vi "UartHelper.vi"() -> ()   [LabVIEW 2012]
uses:
  <vilib>/Platform/TimedLoop/XDataNode/timing_clust.ctl
  <vilib>/Platform/TimedLoop/XDataNode/nitl_modes.ctl
  <vilib>/Platform/TimedLoop/XDataNode/wakeup.ctl
  <vilib>/event_ctls.llb/eventvkey.ctl
  <vilib>/Instr/_visa.llb/VISA Configure Serial Port (Instr).vi
  <vilib>/Platform/TimedLoop/XDataNode/XDataNode.xnode
  <vilib>/Platform/TimedLoop/XDataNode/XDNodeRunTimeDep.lvlib
panel:
  out "串口打开?":bool
  out "附加位":string="\r"
  out "文件發送":path=path "E:/ProJect/#034 串口助手/Libs/SubVi/123.txt"
  out "文件接收":path
  in  "复位计数":bool
  in  "接收计数":u32
  in  "发送计数":u32
  in  "发送数据":bool
  in  "数据发送":string
  in  "数据接收":string
  in  "清除发送":bool
  in  "清除接收":bool
  in  "循环周期":u32
  in  "循环发送":bool
  in  "文件数据源":bool
  in  "自动附加位":bool
  in  "发送模式":enum32{"ASCII", "HEX"}(radio)
  in  "接收模式":enum32{"ASCII", "HEX"}(radio)
  in  "暂停显示":bool
  in  "文件接收":bool
  in  "接收换行":bool
  in  "日志模式":bool
  in  "停止位":u32(ring)=10 items=["1"=10, "1.5"=15, "2"=20]
  in  "校验位":u16(ring) items=["None", "Odd", "Even", "Mark", "Space"]
  in  "数据位":u16(ring)=8 items=["5"=5, "6"=6, "7"=7, "8"=8]
  in  "波特率":u32(ring)=9600 items=["110"=110, "300"=300, "600"=600, "1200"=1200, "2400"=2400, "4800"=4800, "9600"=9600, "14400"=14400, "19200"=19200, "38400"=38400, "56000"=56000, "57600"=527600, "115200"=115200, "128000"=128000, "256000"=256000]
  in  "串口号":refnum<visa-resource-name>="COM1"
  in  "打开串口":bool
  # "串口设置"
  # "接收设置"
  # "发送设置"
  # "ms"
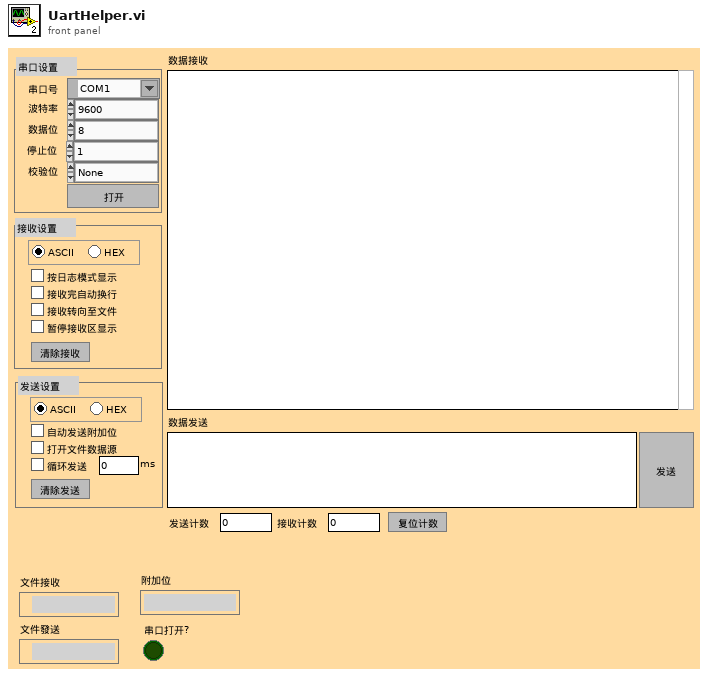
[diagram p1: front panel]
types:
  T1 = typedef "XDNodeRunTimeDep.lvlib/timing_clust.ctl" = cluster{"Expected End [f-1]":u64, "Actual End [f-1]":u64, "Finished Late? [f-1]":bool, "Expected End [i-1]":u64, "Actual End [i-1]":u64, "Finished Late? [i-1]":bool, "Expected Start [i]":u64, "Actual Start [i]":u64, "Expected Start [f]":u64, "Actual Start [f]":u64, "Source Name":string, "Structure Name":string, "Period":i64, "Deadline":i64, "Offset":i64, "Start":i64, "Priority":i32, "Timeout":i32, "Mode":T2, "Wakeup Reason":T3, "Error":errorcluster, "Source Type":string, "Secondary Source Type":string, "Global End Time":u64, "Global Start Time":u64, "Frame Duration":u64, "Iteration Duration":u64, "Assigned CPU":i32, "I/O Scan Engine Mode":u32}
  T2 = typedef "XDNodeRunTimeDep.lvlib/nitl_modes.ctl" = enum32{"No Change", "Process missed periods, maintain original phase", "Discard missed periods, maintain original phase", "Process missed periods, ignore original phase", "Discard missed periods, ignore original phase"}
  T3 = typedef "XDNodeRunTimeDep.lvlib/wakeup.ctl" = enum32{"Normal", "Aborted", "Asynchronous wakeup", "Timing source error", "Timed loop error", "Timeout"}
  T4 = enum8{"Enabled", "Disabled", "Disabled and Grayed Out"}
  T5 = typedef "eventvkey.ctl" = enum16{"ASCII", "Enter", "Return", "Shift", "Ctrl", "Alt", "Cmd", "Opt", "Caps", "NumLock", "Clear", "Break", "Up", "Down", "Left", "Right", "Insert", "Delete", "Home", "End", "PageUp", "PageDown", "Escape", "Help", "Pause", "ScrollLock", "F1", "F2", "F3", "F4", "F5", "F6", "F7", "F8", "F9", "F10", "F11", "F12", "F13", "F14", "F15", "F16", "F17", "F18", "F19", "F20", "F21", "F22", "F23", "F24", "Play", "VolumeUp", "VolumeDown", "Mute", "Two Byte Char"}
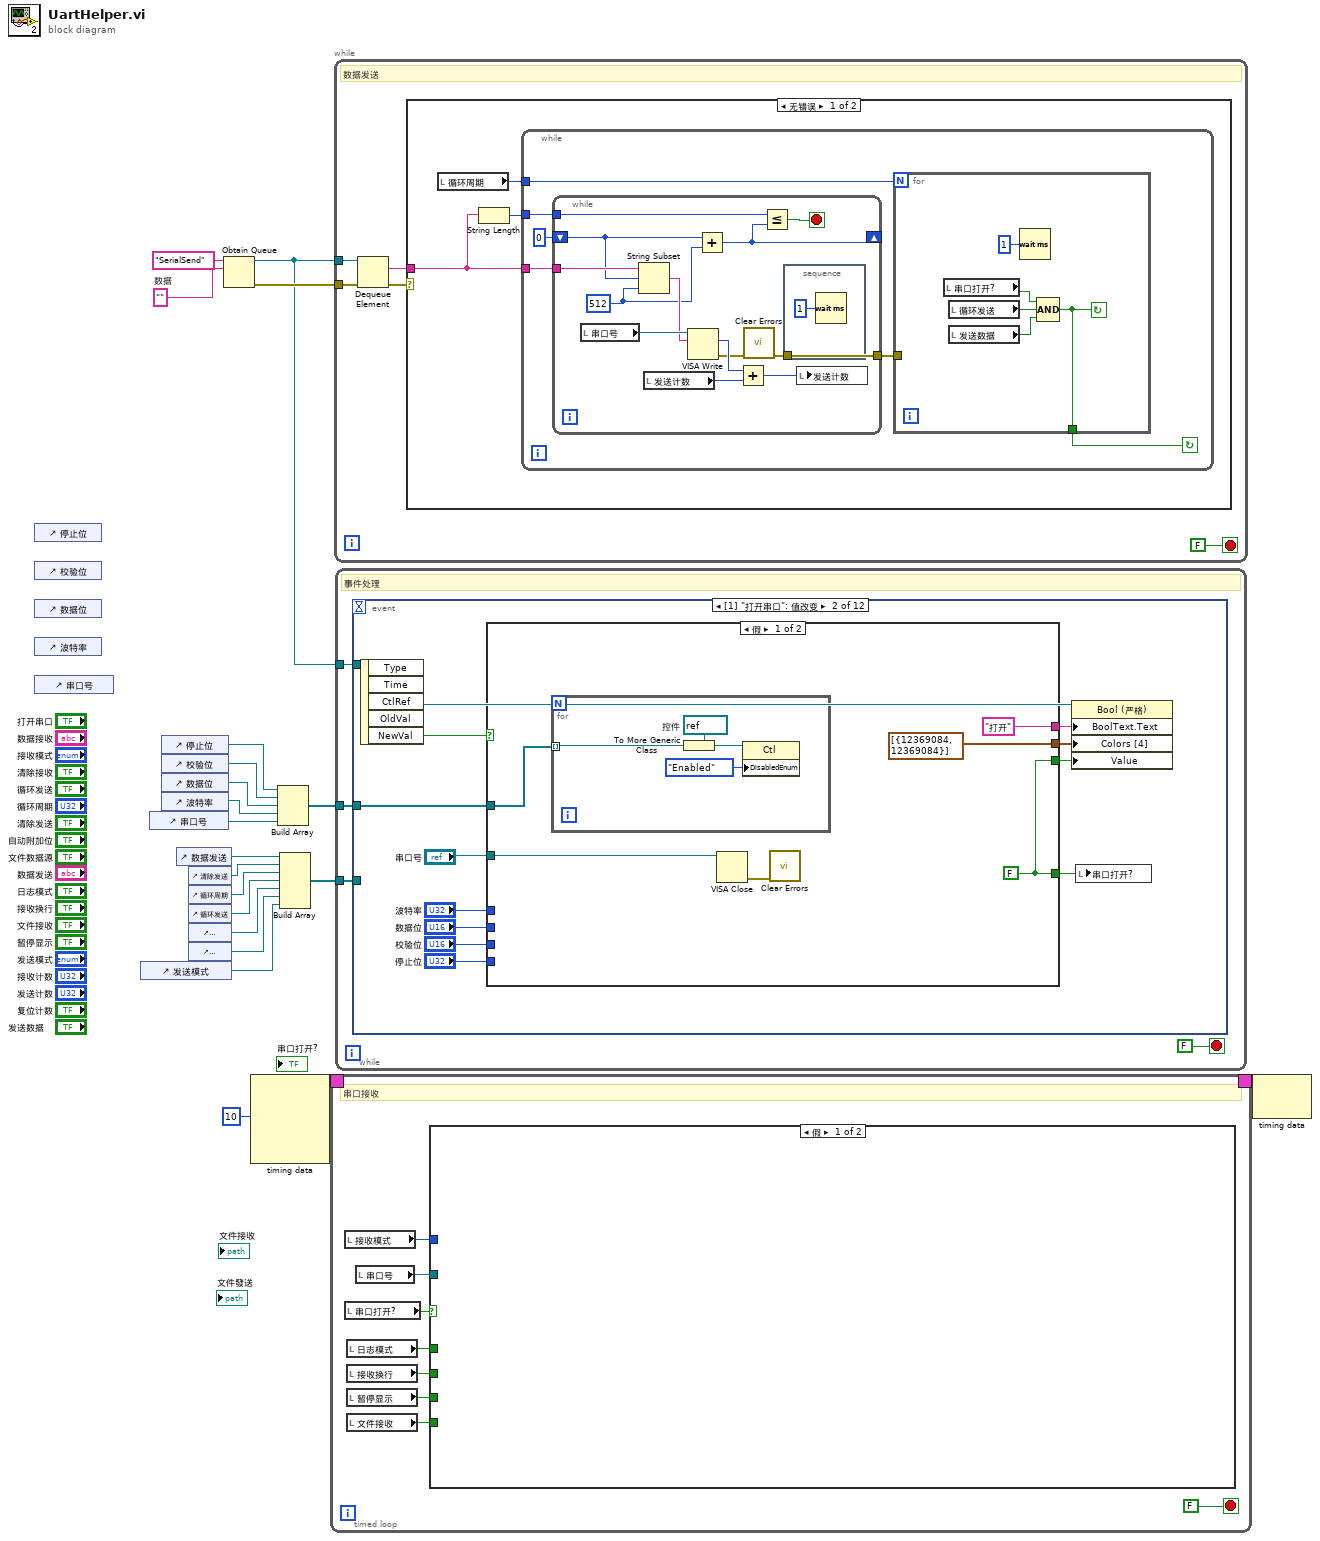
[diagram p0: block diagram]
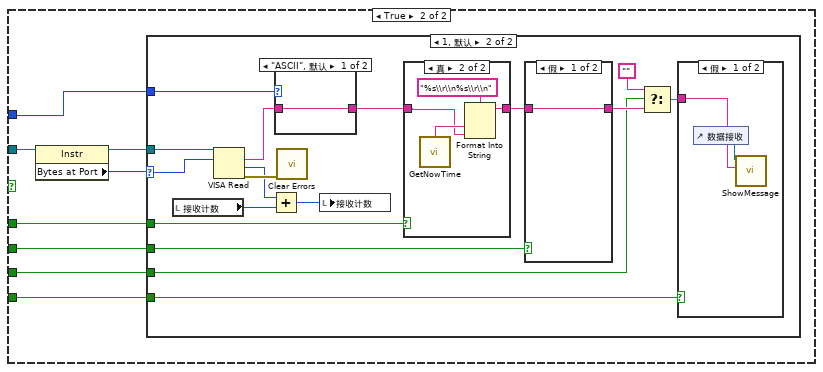
[diagram p3: hidden frame]
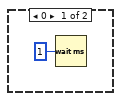
[diagram p4: hidden frame]
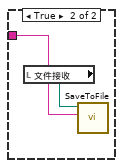
[diagram p5: hidden frame]
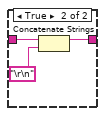
[diagram p6: hidden frame]
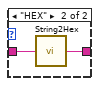
[diagram p8: hidden frame]
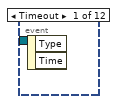
[diagram p9: hidden frame]
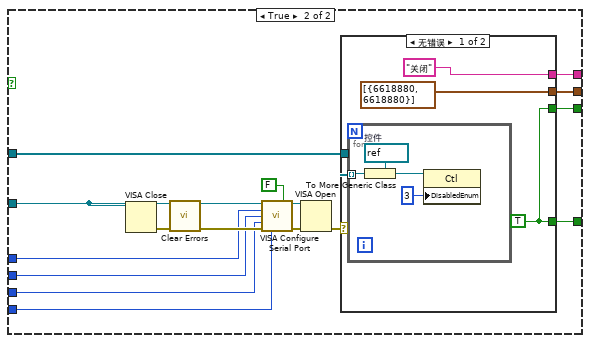
[diagram p10: hidden frame]
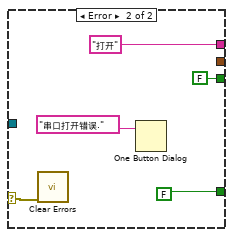
[diagram p11: hidden frame]
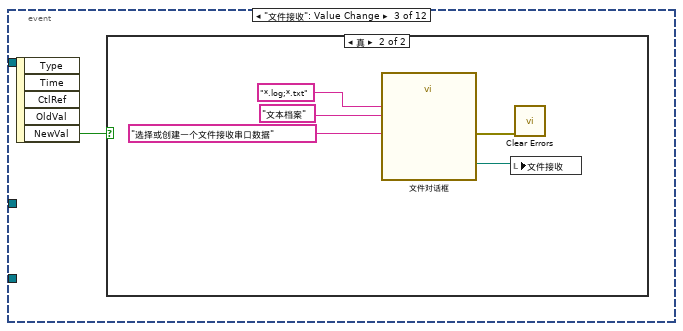
[diagram p12: hidden frame]
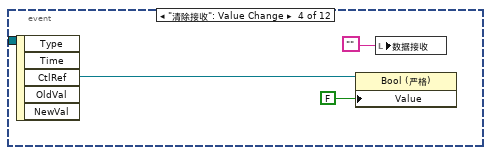
[diagram p14: hidden frame]
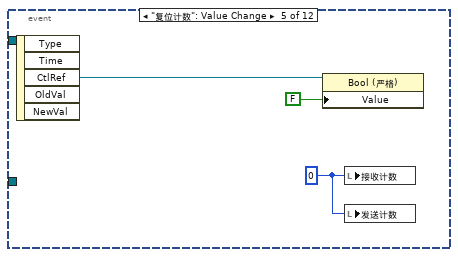
[diagram p15: hidden frame]
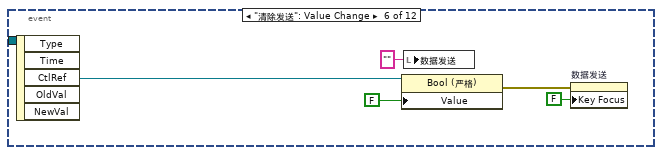
[diagram p16: hidden frame]
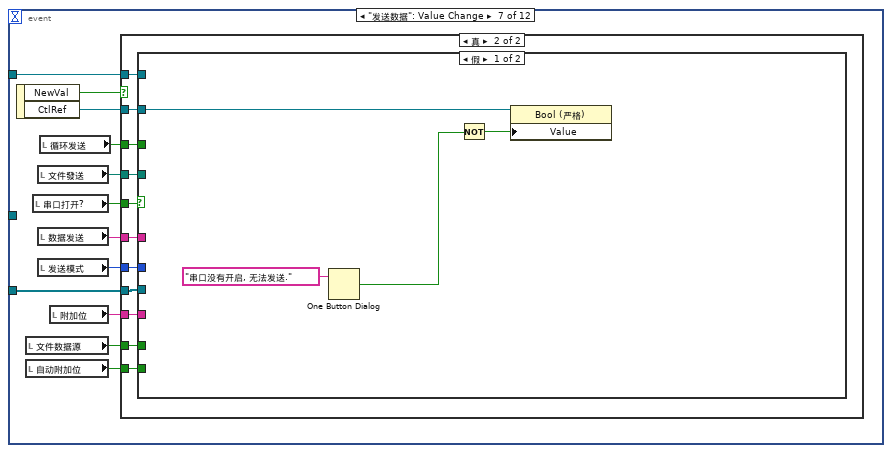
[diagram p17: hidden frame]
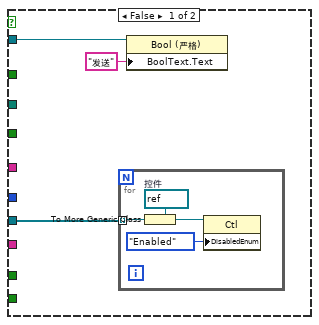
[diagram p18: hidden frame]
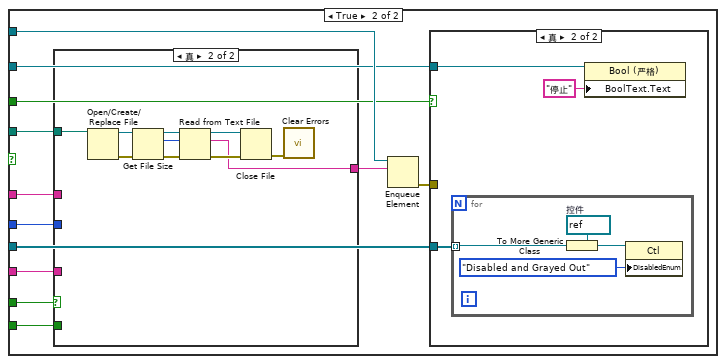
[diagram p19: hidden frame]
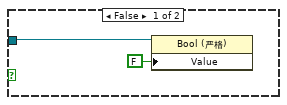
[diagram p20: hidden frame]
diagram:
  w16 = ""  # 数据
  n1 = control-ref of="停止位"() -> ()  [unwired: 1 out]
  n2 = control-ref of="校验位"() -> ()  [unwired: 1 out]
  n3 = control-ref of="数据位"() -> ()  [unwired: 1 out]
  n4 = control-ref of="波特率"() -> ()  [unwired: 1 out]
  n5 = control-ref of="串口号"() -> ()  [unwired: 1 out]
  n6 = control-ref of="发送模式"() -> (w8:refnum<vi>)
  n7 = control-ref of="串口号"() -> (w6:refnum<vi>)
  n8 = control-ref of="停止位"() -> (w2:refnum<vi>)
  n9 = control-ref of="校验位"() -> (w3:refnum<vi>)
  n10 = control-ref of="数据位"() -> (w4:refnum<vi>)
  n11 = control-ref of="波特率"() -> (w5:refnum<vi>)
  n12 = control-ref of="数据发送"() -> (w14:refnum<vi>)
  n13 = control-ref of="清除发送"() -> (w13:refnum<vi>)
  n14 = control-ref of="循环周期"() -> (w12:refnum<vi>)
  n15 = control-ref of="循环发送"() -> (w11:refnum<vi>)
  n16 = control-ref of="文件数据源"() -> (w10:refnum<vi>)
  n17 = control-ref of="自动附加位"() -> (w9:refnum<vi>)
  n18 = Obtain Queue(name (unnamed)="SerialSend" ("名称（未命名）"), element data type=w16) -> (queue out=w15:refnum<queue>, error out=w18:errorcluster)  [unwired: 3 in, 1 out]
  n19 = node-c288(i64 10 ("周期")) -> (w21:T1)  [unwired: 3 in]
  n20 = Build Array(w2, w3, w4, w5, w6) -> (w1:refnum<vi>[])
  n21 = Build Array(w14, w13, w12, w11, w10, w9, w8) -> (w7:refnum<vi>[])
  n22 = timed-loop "接收" {
    timing: w21 -> [_]
    timing-out: [_] -> w20
    stop <- FALSE stop-if-true
    # "串口接收"
    n23 = local read "接收模式"() -> (w27:enum32{"ASCII", "HEX"})
    n24 = local read "串口打开?"() -> (w26:bool)
    n25 = local read "日志模式"() -> (w25:bool)
    n26 = local read "接收换行"() -> (w24:bool)
    n27 = local read "暂停显示"() -> (w23:bool)
    n28 = local read "文件接收"() -> (w22:bool)
    n29 = local read "串口号"() -> (w28:refnum<visa-resource-name>)
    n30 = case shown="假" w26 {
      tunnel: w28 -> [_ w37]
      tunnel: w27 -> [_ w35]
      tunnel: w25 -> [_ w34]
      tunnel: w24 -> [_ w33]
      tunnel: w23 -> [_ w32]
      tunnel: w22 -> [_ w31]
      frame False {
      }
      frame True {
        n31 = property class="Instr"(reference=w37) -> (reference out=w36:refnum<visa-resource-name>, "Bytes at Port"=w30:u32)  [unwired: 1 in, 1 out]
        n32 = case shown="1, 默认" w30 {
          selector: w30 -> [_ w39]
          tunnel: w36 -> [_ w55]
          tunnel: w35 -> [_ w54]
          tunnel: w34 -> [_ w48]
          tunnel: w33 -> [_ w46]
          tunnel: w32 -> [_ w43]
          tunnel: w31 -> [_ w41]
          frame 0 {
            n33 = Wait (ms)(milliseconds to wait=u32 1 ("等待时间（毫秒）")) -> ()  [unwired: 1 out]
          }
          frame 1, Default {
            n34 = local read "接收计数"() -> (w50:u32)
            n35 = VISA Read(VISA resource name=w55, byte count=w39) -> (read buffer=w53:string, return count=w51:u32, error out=w52:errorcluster)  [unwired: 1 in, 1 out]
            n36 = Add(x=w51, y=w50) -> (x+y=w49:u32)
            n37 = case shown="\"ASCII\", 默认" w54 {
              tunnel: w53 -> [w69 w71]
              tunnel: [w69 w70] -> w47
              frame "ASCII", Default {
              }
              frame "HEX" {
                n38 = call "String2Hex.vi"("String"=w71) -> ("Hex"=w70:string)
              }
            }
            n39 = call <vilib>:"Clear Errors.vi"("error in (no error)"=w52) -> ()  [unwired: 6 in, 1 out]
            n40 = local write "接收计数"(w49) -> ()
            n41 = case shown="真" w48 {
              tunnel: w47 -> [w64 w66]
              tunnel: [w64 w68] -> w45
              frame False {
              }
              frame True {
                n42 = call "GetNowTime.vi"() -> ("NowTime"=w67:string)
                n43 = Format Into String(format string="%s\\r\\n%s\\r\\n" ("格式字符串"), w67, w66) -> (resulting string=w68:string)  [unwired: 2 in, 1 out]
              }
            }
            n44 = case shown="假" w46 {
              tunnel: w45 -> [w60 w63]
              tunnel: [w60 w61] -> w44
              frame False {
              }
              frame True {
                n45 = Concatenate Strings(w63, "\r\n") -> (w61:string)
              }
            }
            n46 = Select(t="", s=w43, f=w44) -> (s? t:f=w40:string)
            n47 = case shown="假" w41 {
              tunnel: w40 -> [w56 w59]
              frame False {
                n48 = control-ref of="数据接收"() -> (w57:refnum<vi>)
                n49 = call "ShowMessage.vi"("字符串"=w56, "Str引用句柄"=w57) -> ()  [unwired: 10 in]
              }
              frame True {
                n50 = local read "文件接收"() -> (w58:path)
                n51 = call "SaveToFile.vi"("字符串"=w59, "路径"=w58) -> ()  [unwired: 10 in]
              }
            }
          }
        }
      }
    }
  }
  n52 = while {
    tunnel: w15 -> [w75]
    tunnel: w18 -> [w74]
    stop <- FALSE stop-if-true
    # "数据发送"
    n53 = Dequeue Element(queue=w75, error in (no error)=w74) -> (element=w76:string, error out=w77:errorcluster)  [unwired: 1 in, 2 out]
    n54 = case shown="无错误" w77 {
      tunnel: w76 -> [w80 _]
      frame No Error {
        n55 = local read "循环周期"() -> (w81:u32)
        n56 = String Length(string=w80) -> (length=w79:i32)
        n57 = while {
          tunnel: w80 -> [w87]
          tunnel: w81 -> [w86]
          tunnel: w79 -> [w82]
          stop <- w84 continue-if-true
          n58 = while {
            tunnel: [w88] -> w85
            tunnel: w87 -> [w95]
            shift-right: [w90] -> _
            shift-left: 0 -> [w93]
            tunnel: w82 -> [w91]
            stop <- w89 stop-if-true
            w92 = 512 ("长度（剩余）")
            n59 = local read "串口号"() -> (w100:refnum<visa-resource-name>)
            n60 = String Subset(string=w95, offset (0)=w93, length (rest)=w92) -> (substring=w94:string)
            n61 = local read "发送计数"() -> (w99:u32)
            n62 = VISA Write(VISA resource name=w100, write buffer=w94) -> (return count=w98:u32, error out=w97:errorcluster)  [unwired: 1 in, 1 out]
            n63 = Add(x=w93, y=w92) -> (x+y=w90:i32)
            n64 = Add(x=w98, y=w99) -> (x+y=w96:u32)
            n65 = call <vilib>:"Clear Errors.vi"("error in (no error)"=w97) -> ("error out"=w88:errorcluster)  [unwired: 6 in]
            n66 = Less Or Equal?(x=w91, y=w90) -> (x <= y?=w89:bool)
            n67 = stacked-sequence {
              tunnel: w88 -> [_]
              frame #0 {
                n68 = Wait (ms)(milliseconds to wait=u32 1 ("等待时间（毫秒）")) -> ()  [unwired: 1 out]
              }
            }
            n69 = local write "发送计数"(w96) -> ()
          }
          n70 = for {
            N: w86 -> [_]
            tunnel: w85 -> [_]
            tunnel: [w103] -> w84
            stop <- w103 continue-if-true
            n71 = local read "串口打开?"() -> (w102:bool)
            n72 = local read "循环发送"() -> (w105:bool)
            n73 = local read "发送数据"() -> (w104:bool)
            n74 = Wait (ms)(milliseconds to wait=u32 1 ("等待时间（毫秒）")) -> ()  [unwired: 1 out]
            n75 = Compound Arithmetic op=AND(w102, w105, w104) -> (w103:bool)
          }
        }
      }
      frame Error {
      }
    }
  }
  n76 = while {
    tunnel: w15 -> [w109]
    tunnel: w7 -> [w108]
    tunnel: w1 -> [w107]
    stop <- FALSE stop-if-true
    # "事件处理"
    n77 = event shown="[1] \"打开串口\": 值改变" {
      selector: _ -> [_ _ _ _ _ _ _ _ _ _ _ _]
      dyn-events: _ -> [_ _ _ _ _ _ _ _ _ _ _ _]
      timeout: _ -> [_ _ _ _ _ _ _ _ _ _ _ _]
      tunnel: w109 -> [_ _ _ _ _ _ w185 _ _ _ _ _]
      tunnel: w108 -> [_ _ _ _ _ _ w179 _ _ _ _ _]
      tunnel: w107 -> [_ w116 _ _ _ _ _ _ _ _ _ _]
      event Timeout {
        n78 = event-data() -> ()  [unwired: 1 in, 2 out]
      }
      event "打开串口": Value Change {
        n79 = event-data() -> ("CtlRef"=w121:refnum<vi>, "NewVal"=w122:bool)  [unwired: 1 in, 3 out]
        n80 = case shown="假" w122 {
          tunnel: ["打开" w148] -> w120
          tunnel: [cluster{u32, u32}[] [{12369084, 12369084}] w147] -> w119
          tunnel: [w125 w145] -> w118
          tunnel: [w125 w144] -> w117
          tunnel: w116 -> [w124 w143]
          tunnel: "串口号" -> [w123 w133]
          tunnel: "波特率" -> [_ w140]
          tunnel: "数据位" -> [_ w138]
          tunnel: "校验位" -> [_ w137]
          tunnel: "停止位" -> [_ w136]
          frame False {
            w125 = FALSE
            n81 = for {
              tunnel: w124 -> [w132] mode=indexing
              w131 = refnum<vi> refnum  # 控件
              n82 = To More Generic Class(target class=w131, reference=w132) -> (generic class reference=w130:refnum<vi>)
              n83 = property class="Ctl"(reference=w130, "DisabledEnum"=T4."Enabled" ("禁用")) -> ()  [unwired: 1 in, 2 out]
            }
            n84 = VISA Close(VISA resource name=w123) -> (error out=w126:errorcluster)  [unwired: 1 in]
            n85 = call <vilib>:"Clear Errors.vi"("error in (no error)"=w126) -> ()  [unwired: 6 in, 1 out]
          }
          frame True {
            n86 = VISA Close(VISA resource name=w133) -> (error out=w134:errorcluster)  [unwired: 1 in]
            n87 = call <vilib>:"Clear Errors.vi"("error in (no error)"=w134) -> ("error out"=w141:errorcluster)  [unwired: 6 in]
            n88 = call-poly "VISA Configure Serial Port"("VISA resource name"=w133, "Enable Termination\nChar (T)"=FALSE ("Enable Termination\nChar (T)"), "baud rate (9600)"=w140, "data bits (8)"=w138, "parity (0:none)"=w137, "error in (no error)"=w141, "stop bits (10: 1 bit)"=w136) -> ("VISA resource name out"=w135:refnum<visa-resource-name>, "error out"=w142:errorcluster)  [unwired: 7 in]
            n89 = VISA Open(error in (no error)=w142, VISA resource name=w135) -> (error out=w146:errorcluster)  [unwired: 3 in, 1 out]
            n90 = case shown="无错误" w146 {
              selector: w146 -> [_ w160]
              tunnel: ["关闭" "打开"] -> w148
              tunnel: [cluster{u32, u32}[] [{6618880, 6618880}] _] -> w147
              tunnel: [w150 FALSE] -> w145
              tunnel: [w150 FALSE] -> w144
              tunnel: w143 -> [w149 _]
              frame No Error {
                w150 = TRUE
                n91 = for {
                  tunnel: w149 -> [w156] mode=indexing
                  w155 = refnum<vi> refnum  # 控件
                  n92 = To More Generic Class(target class=w155, reference=w156) -> (generic class reference=w154:refnum<vi>)
                  n93 = property class="Ctl"(reference=w154, "DisabledEnum"=3) -> ()  [unwired: 1 in, 2 out]
                }
              }
              frame Error {
                n94 = call <vilib>:"Clear Errors.vi"("error in (no error)"=w160) -> ()  [unwired: 6 in, 1 out]
                n95 = One Button Dialog(message="串口打开错误.") -> ()  [unwired: 1 in, 1 out]
              }
            }
          }
        }
        n96 = property class="Bool (严格)"(reference=w121, "BoolText.Text"=w120, "Colors [4]"=w119, "Value"=w117) -> ()  [unwired: 1 in, 2 out]
        n97 = local write "串口打开?"(w118) -> ()
      }
      event "文件接收": Value Change {
        n98 = event-data() -> ("NewVal"=w162:bool)  [unwired: 1 in, 4 out]
        n99 = case shown="真" w162 {
          frame False {
          }
          frame True {
            n100 = call "文件对话框"("prompt"="选择或创建一个文件接收串口数据", "pattern (all files)"="*.log;*.txt", "pattern label"="文本档案") -> ("selected path"=w167:path, "error out"=w165:errorcluster)  [unwired: 9 in, 2 out]
            n101 = local write "文件接收"(w167) -> ()
            n102 = call <vilib>:"Clear Errors.vi"("error in (no error)"=w165) -> ()  [unwired: 6 in, 1 out]
          }
        }
      }
      event "清除接收": Value Change {
        n103 = event-data() -> ("CtlRef"=w169:refnum<vi>)  [unwired: 1 in, 4 out]
        n104 = property class="Bool (严格)"(reference=w169, "Value"=FALSE) -> ()  [unwired: 1 in, 2 out]
        n105 = local write "数据接收"("") -> ()
      }
      event "复位计数": Value Change {
        w173 = 0
        n106 = event-data() -> ("CtlRef"=w172:refnum<vi>)  [unwired: 1 in, 4 out]
        n107 = property class="Bool (严格)"(reference=w172, "Value"=FALSE) -> ()  [unwired: 1 in, 2 out]
        n108 = local write "接收计数"(w173) -> ()
        n109 = local write "发送计数"(w173) -> ()
      }
      event "清除发送": Value Change {
        n110 = event-data() -> ("CtlRef"=w177:refnum<vi>)  [unwired: 1 in, 4 out]
        n111 = property class="Bool (严格)"(reference=w177, "Value"=FALSE) -> (error out=w175:errorcluster)  [unwired: 1 in, 1 out]
        n112 = local write "数据发送"("" ("数据发送")) -> ()
        n113 = property on="数据发送" class="Str"(error in=w175, "Key Focus"=FALSE ("键选中")) -> ()  [unwired: 1 in, 2 out]
      }
      event "发送数据": Value Change {
        n114 = event-data() -> ("NewVal"=w180:bool, "CtlRef"=w182:refnum<vi>)  [unwired: 1 in]
        n115 = local read "文件数据源"() -> (w184:bool)
        n116 = local read "自动附加位"() -> (w183:bool)
        n117 = local read "串口打开?"() -> (w188:bool)
        n118 = local read "文件發送"() -> (w186:path)
        n119 = local read "数据发送"() -> (w189:string)
        n120 = local read "发送模式"() -> (w190:enum32{"ASCII", "HEX"})
        n121 = local read "循环发送"() -> (w181:bool)
        n122 = local read "附加位"() -> (w187:string)
        n123 = case shown="真" w180 {
          tunnel: w190 -> [_ w208]
          tunnel: w189 -> [_ w207]
          tunnel: w188 -> [_ w206]
          tunnel: w187 -> [_ w205]
          tunnel: w186 -> [_ w204]
          tunnel: w185 -> [_ w203]
          tunnel: w184 -> [_ w202]
          tunnel: w183 -> [_ w201]
          tunnel: w182 -> [w193 w200]
          tunnel: w181 -> [_ w199]
          tunnel: w179 -> [w191 w198]
          frame False {
            n124 = for {
              tunnel: w191 -> [w197] mode=indexing
              w196 = refnum<vi> refnum  # 控件
              n125 = To More Generic Class(target class=w196, reference=w197) -> (generic class reference=w195:refnum<vi>)
              n126 = property class="Ctl"(reference=w195, "DisabledEnum"=T4."Enabled" ("禁用")) -> ()  [unwired: 1 in, 2 out]
            }
            n127 = property class="Bool (严格)"(reference=w193, "BoolText.Text"="发送" ("布尔文本.文本")) -> ()  [unwired: 1 in, 2 out]
          }
          frame True {
            n128 = case shown="假" w206 {
              tunnel: w208 -> [_ w224]
              tunnel: w207 -> [_ w223]
              tunnel: w205 -> [_ w222]
              tunnel: w202 -> [_ w221]
              tunnel: w204 -> [_ w220]
              tunnel: w203 -> [_ w218]
              tunnel: w201 -> [_ w219]
              tunnel: w200 -> [w211 w214]
              tunnel: w199 -> [_ w216]
              tunnel: w198 -> [_ w213]
              frame False {
                n129 = One Button Dialog(message="串口没有开启, 无法发送." ("消息")) -> (true=w209:bool)  [unwired: 1 in]
                n130 = Not(x=w209) -> (.not. x?=w210:bool)
                n131 = property class="Bool (严格)"(reference=w211, "Value"=w210) -> ()  [unwired: 1 in, 2 out]
              }
              frame True {
                n132 = case shown="真" w221 {
                  tunnel: w224 -> [w239 _]
                  tunnel: w223 -> [w238 _]
                  tunnel: w222 -> [w236 _]
                  tunnel: w220 -> [_ w251]
                  tunnel: [w235 w247] -> w217
                  tunnel: w219 -> [w234 _]
                  frame False {
                    n133 = case shown="\"HEX\"" w239 {
                      tunnel: w238 -> [w244 w246]
                      tunnel: [w244 w245] -> w237
                      frame "ASCII", Default {
                      }
                      frame "HEX" {
                        n134 = call "Hex2String.vi"("Hex"=w246) -> ("String"=w245:string)
                      }
                    }
                    n135 = case shown="真" w234 {
                      tunnel: w237 -> [w240 w243]
                      tunnel: w236 -> [_ w242]
                      tunnel: [w240 w241] -> w235
                      frame False {
                      }
                      frame True {
                        n136 = Concatenate Strings(w243, w242) -> (w241:string)
                      }
                    }
                  }
                  frame True {
                    n137 = Open/Create/Replace File(file path (use dialog)=w251) -> (refnum out=w255:refnum<file>, error out=w256:errorcluster)  [unwired: 5 in, 1 out]
                    n138 = Get File Size(file=w255, error in=w256) -> (refnum out=w250:refnum<file>, size (in bytes)=w248:i64, 0:w249:errorcluster)
                    n139 = Read from Text File(file (use dialog)=w250, count=w248, error in=w249) -> (refnum out=w253:refnum<file>, text=w247:string, error out=w254:errorcluster)  [unwired: 1 in, 1 out]
                    n140 = Close File(refnum=w253, error in=w254) -> (error out=w252:errorcluster)  [unwired: 1 out]
                    n141 = call <vilib>:"Clear Errors.vi"("error in (no error)"=w252) -> ()  [unwired: 6 in, 1 out]
                  }
                }
                n142 = Enqueue Element(queue=w218, element=w217) -> (error out=w215:errorcluster)  [unwired: 2 in, 2 out]
                n143 = case shown="真" w216 {
                  tunnel: w214 -> [w226 w229]
                  tunnel: w215 -> [_ _]
                  tunnel: w213 -> [_ w227]
                  frame False {
                    n144 = property class="Bool (严格)"(reference=w226, "Value"=FALSE ("值")) -> ()  [unwired: 1 in, 2 out]
                  }
                  frame True {
                    n145 = for {
                      tunnel: w227 -> [w233] mode=indexing
                      w232 = refnum<vi> refnum  # 控件
                      n146 = To More Generic Class(target class=w232, reference=w233) -> (generic class reference=w231:refnum<vi>)
                      n147 = property class="Ctl"(reference=w231, "DisabledEnum"=T4."Disabled and Grayed Out" ("禁用")) -> ()  [unwired: 1 in, 2 out]
                    }
                    n148 = property class="Bool (严格)"(reference=w229, "BoolText.Text"="停止" ("布尔文本.文本")) -> ()  [unwired: 1 in, 2 out]
                  }
                }
              }
            }
          }
        }
      }
      event "文件数据源": Value Change {
        n149 = event-data() -> ("CtlRef"=w257:refnum<vi>, "NewVal"=w258:bool)  [unwired: 1 in, 3 out]
        n150 = case shown="假" w258 {
          tunnel: w257 -> [_ w260]
          frame False {
            n151 = property on="数据发送" class="Str"("DisabledEnum"=T4."Enabled" ("禁用")) -> ()  [unwired: 2 in, 2 out]
          }
          frame True {
            n152 = call "文件对话框2"("prompt"="选择一个文件进行发送.") -> ("selected path"=w261:path, "exists"=w262:bool, "error out"=w263:errorcluster)  [unwired: 11 in, 1 out]
            n153 = case shown="无错误" w263 {
              selector: w263 -> [_ w272]
              tunnel: w262 -> [w267 _]
              tunnel: w261 -> [w266 _]
              tunnel: w260 -> [w265 _]
              frame No Error {
                n154 = case shown="真" w267 {
                  selector: w267 -> [w268 _]
                  tunnel: w266 -> [_ w271]
                  tunnel: w265 -> [w269 _]
                  frame False {
                    n155 = property class="Bool (严格)"(reference=w269, "Value"=w268) -> ()  [unwired: 1 in, 2 out]
                  }
                  frame True {
                    n156 = local write "文件發送"(w271) -> ()
                    n157 = property on="数据发送" class="Str"("DisabledEnum"=T4."Disabled and Grayed Out" ("禁用")) -> ()  [unwired: 2 in, 2 out]
                  }
                }
              }
              frame Error {
                n158 = call <vilib>:"Clear Errors.vi"("error in (no error)"=w272) -> ()  [unwired: 6 in, 1 out]
              }
            }
          }
        }
      }
      event "自动附加位": Value Change {
        n159 = event-data() -> ("NewVal"=w273:bool)  [unwired: 1 in, 4 out]
        n160 = case shown="真" w273 {
          frame False {
          }
          frame True {
            n161 = call "AddMessage.vi"() -> ("字符串"=→"附加位":string)
          }
        }
      }
      event "发送模式": Value Change {
        n162 = event-data() -> ("NewVal"=w277:enum32{"ASCII", "HEX"})  [unwired: 1 in, 4 out]
        n163 = local read "数据发送"() -> (w276:string)
        n164 = case shown="\"HEX\"" w277 {
          tunnel: w276 -> [w279 w281]
          tunnel: [w278 w280] -> w275
          frame "ASCII", Default {
            n165 = call "Hex2String.vi"("Hex"=w279) -> ("String"=w278:string)
          }
          frame "HEX" {
            n166 = call "String2Hex.vi"("String"=w281) -> ("Hex"=w280:string)
          }
        }
        n167 = local write "数据发送"(w275) -> ()
      }
      event "数据发送": Key Down? {
        # "输入过滤, 当HEX模式时无法输入十六进制以外的字符"
        n168 = event-data() -> ("Char"=w286:i16, "VKey"=w284:T5)  [unwired: 1 in, 7 out]
        n169 = local read "发送模式"() -> (w282:enum32{"ASCII", "HEX"})
        n170 = case shown="\"ASCII\", 默认" w282 {
          tunnel: w286 -> [w288 w304]
          tunnel: [FALSE w298] -> w285
          tunnel: w284 -> [_ w296]
          tunnel: [w288 w291] -> w283
          frame "ASCII", Default {
          }
          frame "HEX" {
            n171 = To Upper Case(1:w304) -> (0:w291:i16)
            n172 = In Range and Coerce(upper limit=i16 57 ("上限"), x=w291, lower limit=i16 48 ("下限")) -> (In Range?=w300:bool)  [unwired: 1 out]
            n173 = In Range and Coerce(upper limit=i16 70 ("上限"), x=w291, lower limit=i16 65 ("下限")) -> (In Range?=w299:bool)  [unwired: 1 out]
            n174 = Search 1D Array(1D array=i32[] [8, 32], element=w291) -> (index of element=w290:i32)  [unwired: 1 in]
            n175 = Greater Or Equal To 0?(x=w290) -> (x >= 0?=w289:bool)
            n176 = Not Equal?(x=w296, y=eventvkey."ASCII") -> (x != y?=w294:bool)
            n177 = Compound Arithmetic op=OR(w294, w300, w299, w289) -> (w293:bool)
            n178 = Not(x=w293) -> (.not. x?=w298:bool)
          }
        }
        n179 = event-data("Char"=w283, "VKey"=w284, "Discard?"=w285) -> ()  [unwired: 4 in, 1 out]
      }
      event "数据发送": Value Change {
        # "实现的功能, 每键入2个字符可自动添加空格."
        n180 = event-data() -> ("CtlRef"=w308:refnum<vi>, "OldVal"=w307:string, "NewVal"=w306:string)  [unwired: 1 in, 2 out]
        n181 = local read "发送模式"() -> (w305:enum32{"ASCII", "HEX"})
        n182 = case shown="\"HEX\"" w305 {
          tunnel: w308 -> [_ w314]
          tunnel: w307 -> [_ w313]
          tunnel: w306 -> [_ w312]
          frame "ASCII", Default {
          }
          frame "HEX" {
            n183 = String Length(string=w312) -> (length=w311:i32)
            n184 = String Length(string=w313) -> (length=w310:i32)
            n185 = Less?(x=w311, y=w310) -> (x < y?=w309:bool)
            n186 = case shown="假" w309 {
              tunnel: w314 -> [w320 _]
              tunnel: w312 -> [w317 _]
              frame False {
                n187 = call <vilib>:"Space Constant.vi"() -> ("String"=w319:string)
                n188 = Search and Replace String(replace all?=TRUE ("替换全部？(F)"), input string=w317, search string=w319, replace string="") -> (result string=w321:string)  [unwired: 4 in, 3 out]
                n189 = String Length(string=w321) -> (length=w315:i32)
                n190 = Greater Than 0?(x=w315) -> (x > 0?=w316:bool)
                n191 = case shown="真" w316 {
                  tunnel: w315 -> [_ w328]
                  tunnel: w320 -> [_ w325]
                  frame False {
                  }
                  frame True {
                    n192 = Quotient & Remainder(x=w328, y=2) -> (x-y*floor(x/y)=w327:i32)  [unwired: 1 out]
                    n193 = Equal?(x=0, y=w327) -> (x = y?=w324:bool)
                    n194 = case shown="真" w324 {
                      tunnel: w325 -> [_ w334]
                      frame False {
                      }
                      frame True {
                        n195 = property class="Str"(reference=w334) -> (reference out=w331:refnum<vi>, "Text.Text"=w333:string)  [unwired: 1 in, 1 out]
                        n196 = Concatenate Strings(w333, " " ("字符串")) -> (w329:string)
                        n197 = String Length(string=w329) -> (length=w330:i32)
                        n198 = property class="Str"(reference=w331, "Text.Text"=w329, "Text.Selection Start"=w330) -> ()  [unwired: 1 in, 2 out]
                      }
                    }
                  }
                }
              }
              frame True {
              }
            }
          }
        }
      }
    }
  }
  n199 = node-c288(w20) -> ()  [unwired: 1 out]
